vi "DrawSprites.vi"(8 "error in (no error)":errorcluster, 10 "RT_Game.lvlib:Game.lvclass":refnum<class "Game.lvclass">, 11 "SpriteHandler in":refnum<class "SpriteHandler.lvclass">) -> (0 "error out":errorcluster, 2 "RT_Game.lvlib:Game.lvclass 2":refnum<class "Game.lvclass">, 3 "SpriteHandler out":refnum<class "SpriteHandler.lvclass">)   [LabVIEW 2019, in "RT_Game.lvlib" / "SpriteHandler.lvclass"]
uses:
  SpriteHandler.lvclass
  Game/Game.lvclass
  Game/Game.lvclass/Game.ctl
  SpriteHandler.lvclass/SpriteHandler.ctl
  FPGA/Sprite/SpriteData.ctl
  GameObject/GameObject.lvclass/GameObject.ctl
  RT_Sprite/RT_Sprite.lvclass/RT_Sprite.ctl
  GameObject/Read position.vi
  GameObject/Read size.vi
  GameObject/Read IsActive.vi
  RT_Sprite/Read TransparentColor.vi
  Game/Read FPGA_ref.vi
  Game/Write FPGA_ref.vi
  RT_Sprite/RT_Sprite.lvclass
  C:/Users/FreshBob/Dropbox/VIs/myRIO_GameConsole/RT/RT_Game/GameObject/GameObject.lvclass
  <vilib>/Utility/error.llb/Error Cluster From Error Code.vi
  <vilib>/rvi/errors/niLvFpgaAdjustHostInterfaceError.vi
  FPGA_Interface.ctl
  <vilib>/rvi/interface/nirviReadWriteControl/nirviReadWriteControl.xnode
  FPGA Bitfiles/myriogameconsole_FPGATarget_Main_ntsPRcBZGxk.lvbitx
  FPGA/Sprite/Sprite.lvlib
  NiFpgaLv.dll
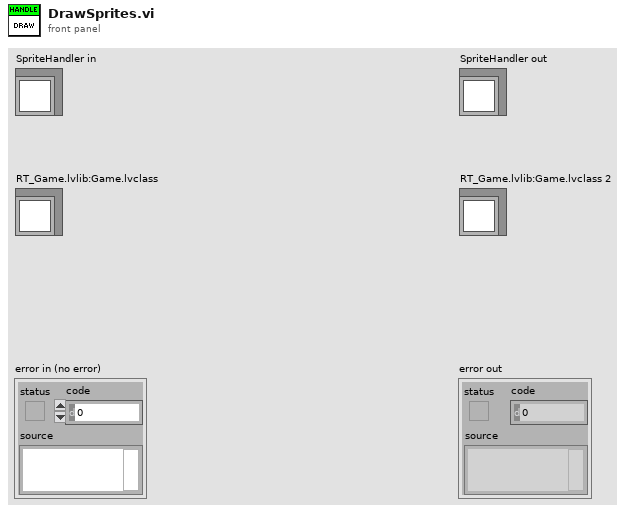
[diagram p1: front panel]
types:
  T1 = typedef "Sprite.lvlib/SpriteData.ctl" = cluster{"Pos_X":u16, "Pos_Y":u16, "Width":u8, "Height":u8, "BufferIndex":u16, "TransparencyColor":fxp<+,3,3>}
  T2 = typedef "RT_Game.lvlib/Game.lvclass/Coordinate.ctl" = cluster{"x":i16, "y":i16}
  T3 = typedef "FPGA_Interface.ctl" = refnum<k20>
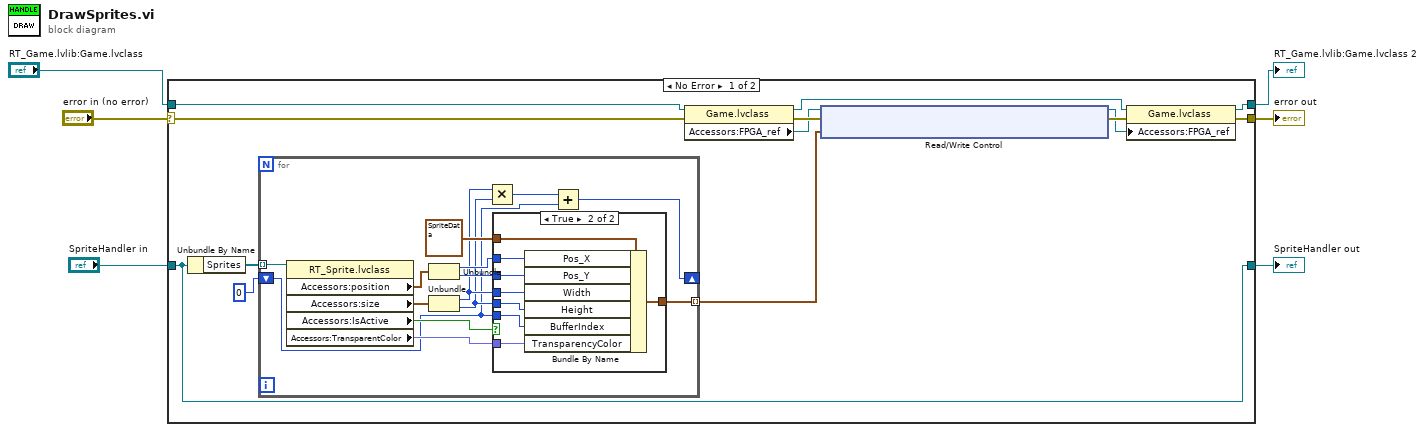
[diagram p0: block diagram]
diagram:
  n1 = case shown="No Error" "error in (no error)" {
    selector: "error in (no error)" -> [w14 w45]
    tunnel: [w15 w45] -> w5
    tunnel: [w9 w44] -> w3
    tunnel: "SpriteHandler in" -> [w9 w44]
    tunnel: [w18 w43] -> w2
    tunnel: "RT_Game.lvlib:Game.lvclass" -> [w19 w43]
    frame No Error {
      n2 = Unbundle By Name(w9) -> ("Sprites"=w8:refnum<class "RT_Sprite.lvclass">[])
      n3 = for {
        tunnel: [w31] -> w10 mode=indexing
        tunnel: w8 -> [w32] mode=indexing
        shift-right: [w24] -> _
        shift-left: u16 0 ("BufferIndex") -> [w20]
        n4 = property class="RT_Sprite.lvclass"(reference=w32) -> ("Accessors:position"=w30:T2, "Accessors:size"=w28:T2, "Accessors:IsActive"=w22:bool, "Accessors:TransparentColor"=w21:fxp<+,3,3>)  [unwired: 1 in, 2 out]
        n5 = Unbundle(w30) -> ("x"=w27:i16, "y"=w29:i16)
        n6 = Unbundle(w28) -> ("x"=w26:i16, "y"=w25:i16)
        n7 = Multiply(x=w26, y=w25) -> (x*y=w23:i16)
        n8 = case shown="True" w22 {
          tunnel: T1 {"Pos_X"=0, "Pos_Y"=0, "Width"=0, "Height"=0, "BufferIndex"=0, "TransparencyColor"=0.0} ("Sprite1") -> [w34 w42]
          tunnel: [w34 w41] -> w31
          tunnel: w29 -> [_ w40]
          tunnel: w27 -> [_ w39]
          tunnel: w26 -> [_ w38]
          tunnel: w25 -> [_ w37]
          tunnel: w21 -> [_ w36]
          tunnel: w20 -> [_ w35]
          frame False {
          }
          frame True {
            n9 = Bundle By Name(cluster=w42, "Pos_X"=w39, "Pos_Y"=w40, "Width"=w38, "Height"=w37, "BufferIndex"=w35, "TransparencyColor"=w36) -> (w41:T1)
          }
        }
        n10 = Add(x=w23, y=w20) -> (x+y=w24:u16)
      }
      n11 = property class="Game.lvclass"(reference=w19, error in=w14) -> (reference out=w17:refnum<class "Game.lvclass">, error out=w16:errorcluster, "Accessors:FPGA_ref"=w12:T3)
      n12 = xnode "Read/Write Control"("FPGA VI Reference In"=w12, "error in"=w16, "Sprites"=w10) -> ("FPGA VI Reference Out"=w11:T3, "error out"=w13:errorcluster)
      n13 = property class="Game.lvclass"(reference=w17, error in=w13, "Accessors:FPGA_ref"=w11) -> (reference out=w18:refnum<class "Game.lvclass">, error out=w15:errorcluster)
    }
    frame Error {
    }
  }
  "error out" <- w5
  "SpriteHandler out" <- w3
  "RT_Game.lvlib:Game.lvclass 2" <- w2
